vi "Get Object ACL.vi"(6 "Version ID":string, 8 "error in (no error)":errorcluster, 10 "Object Key":string, 11 "Bucket in":refnum<class "Bucket.lvclass">) -> (0 "error out":errorcluster, 2 "Access Control Policy":T1, 3 "Bucket out":refnum<class "Bucket.lvclass">)   [LabVIEW 2015, in "NI_AWS_S3.lvlib" / "Bucket.lvclass"]
doc: "This implementation of the GET operation uses the acl subresource to return the access control list (ACL) of an object. To use this operation, you must have READ_ACP access to the object."
uses:
  Bucket.lvclass
  Access Control Policy.ctl
  User.ctl
  Grantee-Permission Pair.ctl
  Permission.ctl
  Core/HTTP Request/Request Options.ctl
  Core/HTTP Request/Name Value Pair.ctl
  Core/HTTP Request/Region handling.ctl
  Core/HTTP Request/URL formatting.ctl
  Bucket.lvclass/Bucket.ctl
  Read Name.vi
  Core/HTTP Request/HTTP Request.lvclass
  NI_AWS_S3.lvlib
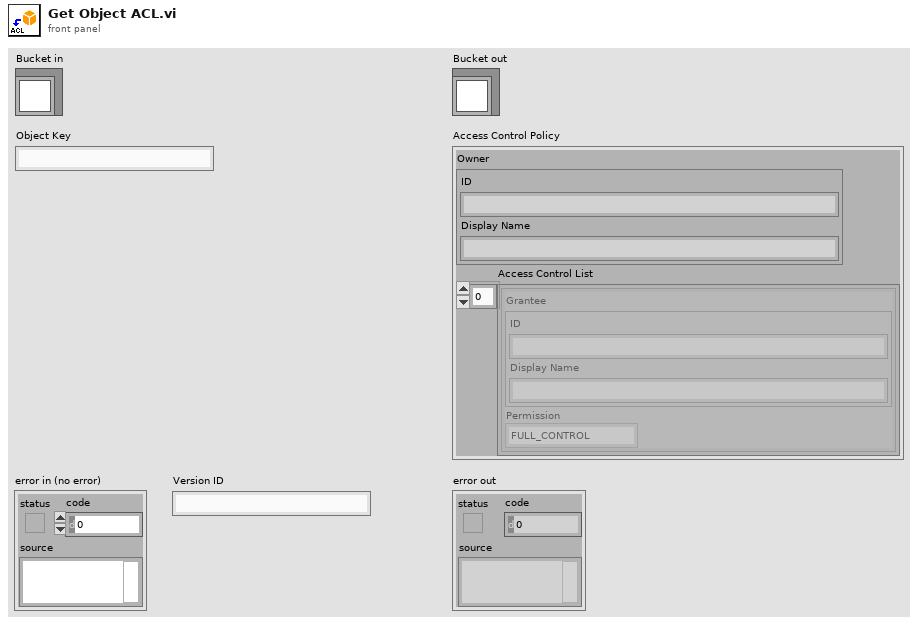
[diagram p1: front panel]
types:
  T1 = typedef "NI_AWS_S3.lvlib/Access Control Policy.ctl" = cluster{"Owner":T2, "Access Control List":T3[]}
  T2 = typedef "NI_AWS_S3.lvlib/User.ctl" = cluster{"ID":string, "Display Name":string}
  T3 = typedef "NI_AWS_S3.lvlib/Grantee-Permission Pair.ctl" = cluster{"Grantee":T2, "Permission":T4}
  T4 = typedef "NI_AWS_S3.lvlib/Permission.ctl" = enum16{"FULL_CONTROL", "WRITE", "WRITE_ACP", "READ", "READ_ACP"}
  T5 = typedef "NI_AWS_Core.lvlib/HTTP Request.lvclass/Name Value Pair.ctl" = cluster{"name":string, "value":string}
  T6 = typedef "NI_AWS_Core.lvlib/HTTP Request.lvclass/Region handling.ctl" = enum16{"use region everywhere", "use region (authentication only)", "use region (URL only)", "ignore region everwhere"}
  T7 = typedef "NI_AWS_Core.lvlib/HTTP Request.lvclass/Request Options.ctl" = cluster{"request headers":T5[], "request parameters":T5[], "request body":string, "region handling":T6, "URL formatting":T8}
  T8 = typedef "NI_AWS_Core.lvlib/HTTP Request.lvclass/URL formatting.ctl" = enum16{"region-", "region."}
  T9 = typedef "NI_AWS_Core.lvlib/HTTP Request.lvclass/Response.ctl" = cluster{"Headers":string, "Body":string}
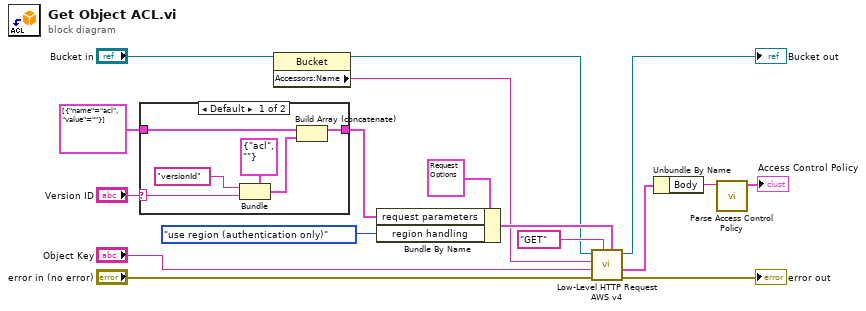
[diagram p0: block diagram]
diagram:
  n1 = case shown="Default" "Version ID" {
    selector: "Version ID" -> [w20 _]
    tunnel: [w21 w24] -> w9
    tunnel: T5[] [{"name"="acl", "value"=""}] ("appended array") -> [w19 w24]
    frame Default {
      n2 = Bundle(cluster=T5 {"name"="acl", "value"=""}, "name"="versionId", "value"=w20) -> (w22:T5)
      n3 = Build Array (concatenate)(w19, w22) -> (w21:T5[])
    }
    frame "" {
    }
  }
  n4 = property class="Bucket"(reference="Bucket in") -> (reference out=w5:refnum<class "Bucket.lvclass">, "Accessors:Name"=w4:string)  [unwired: 1 in, 1 out]
  n5 = Bundle By Name(cluster=T7 {"request headers"=[], "request parameters"=[], "request body"="", "region handling"=enum."use region everywhere", "URL formatting"=enum."region."} ("Request Options"), "request parameters"=w9, "region handling"=Region_handling."use region (authentication only)") -> (w14:T7)
  n6 = call "Low-Level HTTP Request AWS v4.vi"("Request Options"=w14, "HTTP-Verb"="GET", "error in (no error)"="error in (no error)", "URL Suffix"="Object Key", "URL Prefix"=w4, "AWS Core in"=w5) -> ("error out"=→"error out":errorcluster, "Response"=w1:T9, "AWS Core out"=→"Bucket out":refnum<class "Bucket.lvclass">)  [unwired: 2 in, 1 out]
  n7 = Unbundle By Name(w1) -> ("Body"=w3:string)
  n8 = call "Parse Access Control Policy.vi"("Body"=w3) -> ("Access Control Policy"=→"Access Control Policy":T1)  [unwired: 10 in]
